vi "Measure.vi"(8 "error in (no error)":errorcluster, 11 "Experiment3D in":refnum<class "Experiment3D.lvclass">) -> (0 "error out":errorcluster, 2 "End?":bool=TRUE, 3 "Experiment3D out":refnum<class "Experiment3D.lvclass">)   [LabVIEW 2014, in "Experiment3D.lvclass"]
uses:
  Experiment3D.lvclass
  Measurement/Measurement3D/Measurement3D.lvclass
  Data/Data3D/Data3D.lvclass
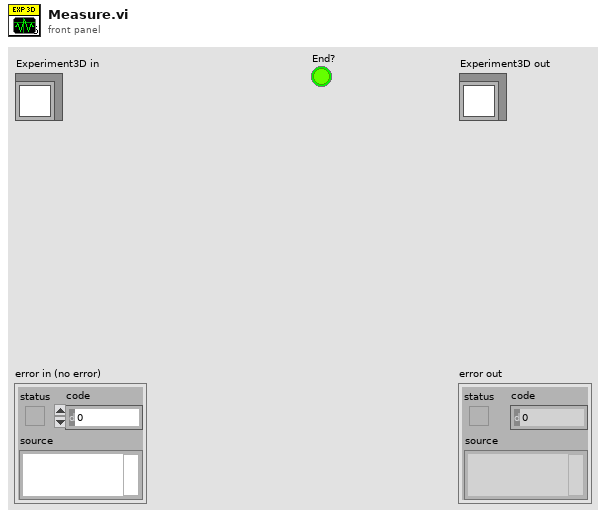
[diagram p1: front panel]
types:
  T1 = cluster{"Init":dbl, "Step":dbl, "Max":dbl, "Current Value":dbl, "Current Index":dbl, "Sweep Outer":dbl[]}
  T2 = cluster{"Init":dbl, "Step":dbl, "Max":dbl, "Current Value":dbl, "Current Index":dbl, "Sweep Inner":dbl[]}
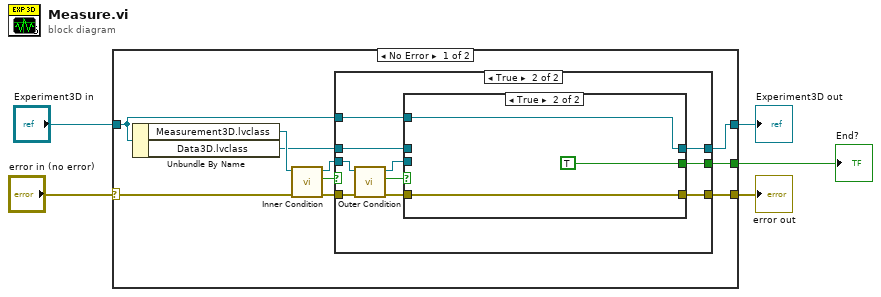
[diagram p0: block diagram]
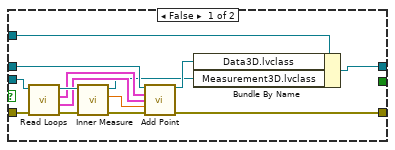
[diagram p2: hidden frame]
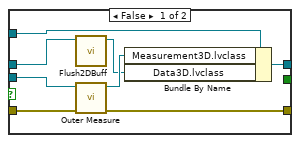
[diagram p3: hidden frame]
diagram:
  n1 = case shown="No Error" "error in (no error)" {
    selector: "error in (no error)" -> [w8 w52]
    tunnel: [w9 w52] -> w4
    tunnel: [w7 w51] -> w2
    tunnel: "Experiment3D in" -> [w12 w51]
    tunnel: [w6 _] -> w1
    frame No Error {
      n2 = Unbundle By Name(w12) -> ("Measurement3D.lvclass"=w15:refnum<class "Measurement3D.lvclass">, "Data3D.lvclass"=w11:refnum<class "Data3D.lvclass">)
      n3 = call "Inner Condition.vi"("error in (no error)"=w8, "Measurement3D in"=w15) -> ("error out"=w10:errorcluster, "Finish?"=w14:bool, "Measurement3D out"=w13:refnum<class "Measurement3D.lvclass">)  [unwired: 7 in]
      n4 = case shown="True" w14 {
        tunnel: w13 -> [w27 w38]
        tunnel: w12 -> [w19 w36]
        tunnel: w11 -> [w23 w31]
        tunnel: w10 -> [w21 w33]
        tunnel: [w29 w35] -> w9
        tunnel: [w17 w32] -> w7
        tunnel: [_ w30] -> w6
        frame False {
          n5 = call "Read Loops.vi"("error in (no error)"=w21, "Measurement3D in"=w27) -> ("error out"=w22:errorcluster, "Outer Loop"=w24:T1, "Inner Loop"=w25:T2, "Measurement3D out"=w26:refnum<class "Measurement3D.lvclass">)  [unwired: 6 in]
          n6 = call "Inner Measure.vi"("error in (no error)"=w22, "Measurement3D in"=w26) -> ("error out"=w20:errorcluster, "Result"=w28:dbl, "Measurement3D out"=w16:refnum<class "Measurement3D.lvclass">)  [unwired: 6 in, 1 out]
          n7 = call "Add Point.vi"("Data3D in"=w23, "Inner Loop"=w25, "Outer Loop"=w24, "Z"=w28, "error in (no error)"=w20) -> ("Data3D out"=w18:refnum<class "Data3D.lvclass">, "error out"=w29:errorcluster)  [unwired: 9 in]
          n8 = Bundle By Name(cluster=w19, "Data3D.lvclass"=w18, "Measurement3D.lvclass"=w16) -> (w17:refnum<class "Experiment3D.lvclass">)
        }
        frame True {
          n9 = call "Outer Condition.vi"("error in (no error)"=w33, "Measurement3D in"=w38) -> ("error out"=w34:errorcluster, "Finish?"=w37:bool, "Measurement3D out"=w39:refnum<class "Measurement3D.lvclass">)  [unwired: 7 in]
          n10 = case shown="True" w37 {
            tunnel: w39 -> [w47 _]
            tunnel: w36 -> [w44 w49]
            tunnel: [w46 w48] -> w35
            tunnel: w34 -> [w45 w48]
            tunnel: [w42 w49] -> w32
            tunnel: w31 -> [w41 _]
            tunnel: [_ TRUE] -> w30
            frame False {
              n11 = call "Flush2DBuff.vi"("Data3D in"=w41) -> ("Data3D out"=w40:refnum<class "Data3D.lvclass">)  [unwired: 9 in, 1 out]
              n12 = call "Outer Measure.vi"("error in (no error)"=w45, "Measurement3D in"=w47) -> ("error out"=w46:errorcluster, "Measurement3D out"=w43:refnum<class "Measurement3D.lvclass">)  [unwired: 7 in, 1 out]
              n13 = Bundle By Name(cluster=w44, "Measurement3D.lvclass"=w43, "Data3D.lvclass"=w40) -> (w42:refnum<class "Experiment3D.lvclass">)
            }
            frame True {
            }
          }
        }
      }
    }
    frame Error {
    }
  }
  "error out" <- w4
  "Experiment3D out" <- w2
  "End?" <- w1
